vi "FCI_Box_Width.vi"(0 "Image In":T9, 1 "Calibrated Image":T9, 2 "OverlayOptions":T5, 3 "Reference Edge ROI":T12 {"Contours"."Type" items=["No Selection", "Point", "Line", "Rectangle", "Oval", "Polygon", "Freehand Region", "Annulus", "Unused2", "Unused3", "Broken Line", "Freehand Line", "Rotated Rectangle"]}, 4 "Blob Center":cluster{"Center X":dbl, "Center Y":dbl}, 5 "Edge Options Ref ROI":T7={"Edge Polarity"=0, "Kernel Size"=3, "Width"=3, "Minimum Edge Strength"=50.0, "Interpolation Type"=enum."Zero Order", "Data Processing Method"=enum."Average"} {"Edge Polarity" items=["All Edges", "Rising Edges", "Falling Edges"]; "Minimum Edge Strength" format="%.2f"; "Width" step=2; "Kernel Size" step=2}, 7 "error in (no error) 2":errorcluster, 8 "Line Options Ref ROI":T10={"Number of Lines"=1, "Type"=enum."First Edge Rake", "Min. Score"=10.0, "Max. Score"=1000.0, "Orientation"=0.0, "Angle Range"=45.0, "Angle Tolerance"=1.0, "Step Size"=3, "Min. SNR (db)"=0.0, "Min. Points (%)"=25.0, "Hough Iterations"=5} {"Min. Points (%)" min=0.0 max=100.0; "Min. SNR (db)" min=0.0; "Max. Score" min=0.0 max=1024.0; "Min. Score" min=0.0 max=1024.0 step=1.0}, 9 "Search Direction Ref ROI":u32=3, 12 "Edge Options ROI 1":T7={"Edge Polarity"=0, "Kernel Size"=5, "Width"=5, "Minimum Edge Strength"=50.0, "Interpolation Type"=enum."Zero Order", "Data Processing Method"=enum."Average"} {"Edge Polarity" items=["All Edges", "Rising Edges", "Falling Edges"]; "Minimum Edge Strength" format="%.2f"; "Width" step=2; "Kernel Size" step=2}, 13 "Step Size ROI 1":u32=2, 14 "Process ROI 1":T6(ring)=enum."Get First + Last Edge", 15 "Scan Direction ROI 1":u16(ring)=2 items=["Left To Right", "Right To Left", "Top To Bottom", "Bottom To Top"]) -> (18 "Overlay Arrow Lines":T1, 20 "Box Edge Information":T4, 21 "Box Width":sgl, 27 "error IO":errorcluster)   [LabVIEW 2019, in "Algorithm.lvclass"]
uses:
  FrameworkOverrides/Algorithm.lvclass
  <vilib>/vision/Measure.llb/Edge Options.ctl
  <vilib>/vision/Measure.llb/Edge Polarity.ctl
  <vilib>/vision/NI_Vision_Development_Module.lvlib
  <vilib>/vision/Measure.llb/Straight Edge Process.ctl
  <vilib>/vision/Measure.llb/Straight Edge Options.ctl
  <vilib>/vision/Image Controls.llb/IMAQ Image.ctl
panel:
  out "Second Overlay Line":T2
  out "First Overlay Line":T3
  out "Angle (Pixel)":dbl
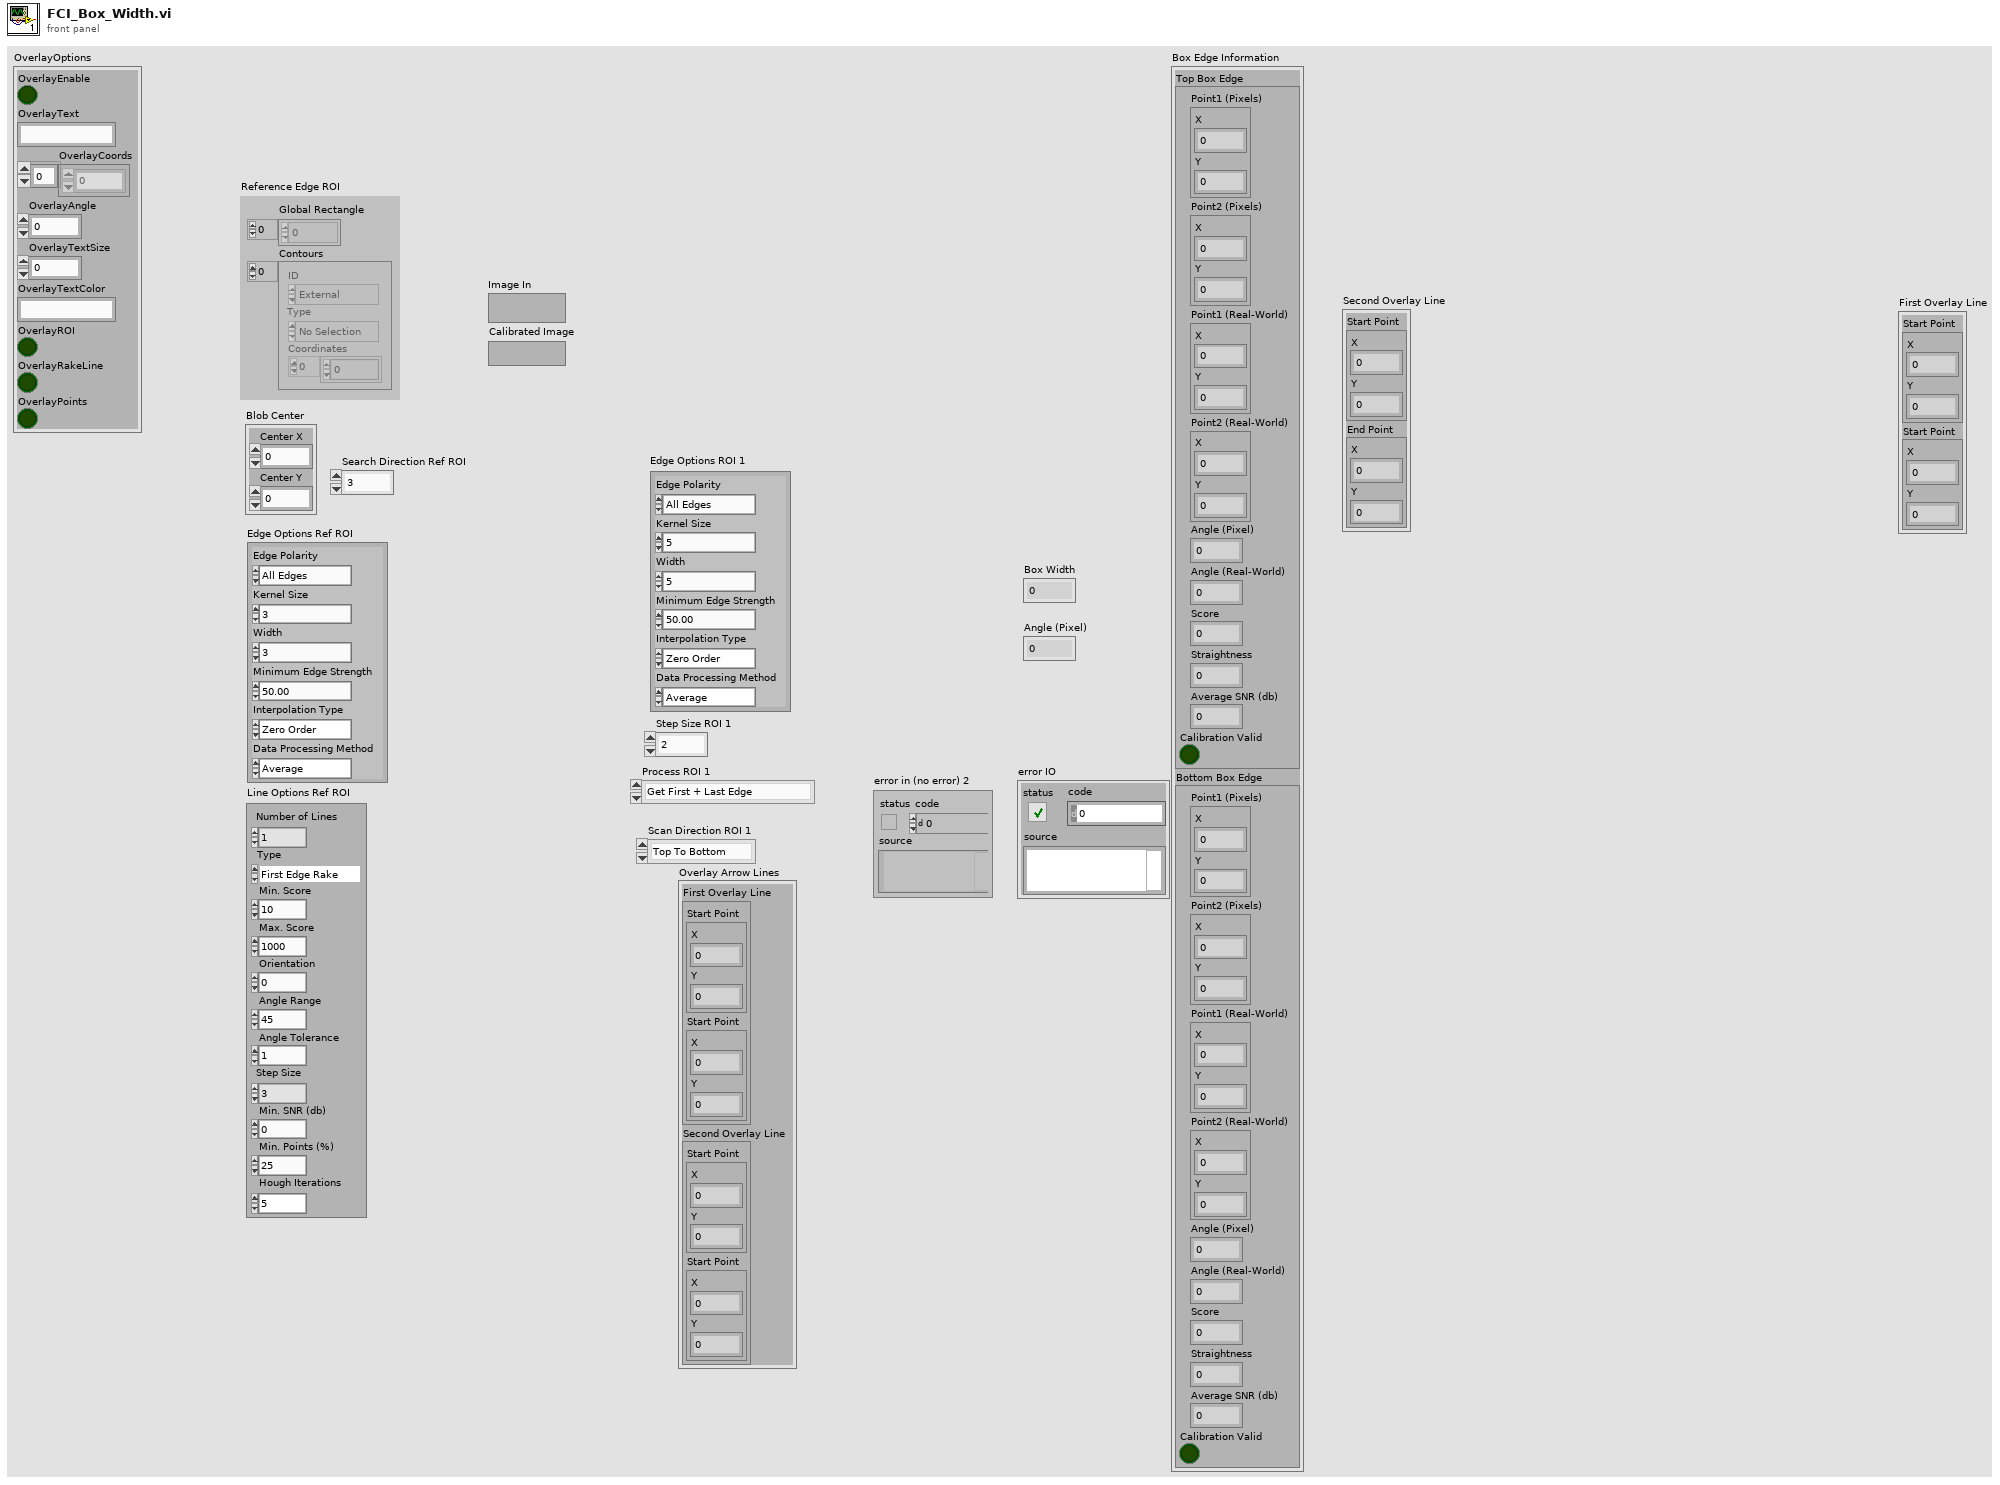
[diagram p1: front panel]
types:
  T1 = cluster{"First Overlay Line ":cluster{"Start Point":cluster{"X":sgl, "Y":sgl}, "Start Point":cluster{"X":sgl, "Y":sgl}}, "Second Overlay Line ":cluster{"Start Point":cluster{"X":sgl, "Y":sgl}, "Start Point":cluster{"X":sgl, "Y":sgl}}}
  T2 = cluster{"Start Point":cluster{"X":sgl, "Y":sgl}, "End Point":cluster{"X":sgl, "Y":sgl}}
  T3 = cluster{"Start Point":cluster{"X":sgl, "Y":sgl}, "Start Point":cluster{"X":sgl, "Y":sgl}}
  T4 = cluster{"Top Box Edge":cluster{"Point1 (Pixels)":cluster{"X":sgl, "Y":sgl}, "Point2 (Pixels)":cluster{"X":sgl, "Y":sgl}, "Point1 (Real-World)":cluster{"X":sgl, "Y":sgl}, "Point2 (Real-World)":cluster{"X":sgl, "Y":sgl}, "Angle (Pixel)":dbl, "Angle (Real-World)":dbl, "Score":dbl, "Straightness":dbl, "Average SNR (db)":dbl, "Calibration Valid":bool}, "Bottom Box Edge":cluster{"Point1 (Pixels)":cluster{"X":sgl, "Y":sgl}, "Point2 (Pixels)":cluster{"X":sgl, "Y":sgl}, "Point1 (Real-World)":cluster{"X":sgl, "Y":sgl}, "Point2 (Real-World)":cluster{"X":sgl, "Y":sgl}, "Angle (Pixel)":dbl, "Angle (Real-World)":dbl, "Score":dbl, "Straightness":dbl, "Average SNR (db)":dbl, "Calibration Valid":bool}}
  T5 = cluster{"OverlayEnable":bool, "OverlayText":string, "OverlayCoords":i32[], "OverlayAngle":i32, "OverlayTextSize":i32, "OverlayTextColor":string, "OverlayROI":bool, "OverlayRakeLine":bool, "OverlayPoints":bool}
  T6 = enum16{"Get First Edge", "Get First + Last Edge", "Get All Edges", "Get Best Edge"}
  T7 = typedef "Edge Options.ctl" = cluster{"Edge Polarity":T8, "Kernel Size":u32, "Width":u32, "Minimum Edge Strength":sgl, "Interpolation Type":enum32{"Zero Order", "Bilinear", "Quadratic", "Cubic", "Bilinear Fixed"}, "Data Processing Method":enum32{"Average", "Median"}}
  T8 = typedef "Edge Polarity.ctl" = u32
  T9 = typedef "IMAQ Image.ctl" = refnum<image>
  T10 = typedef "Straight Edge Options.ctl" = cluster{"Number of Lines":i32, "Type":T11, "Min. Score":dbl, "Max. Score":dbl, "Orientation":dbl, "Angle Range":dbl, "Angle Tolerance":dbl, "Step Size":u32, "Min. SNR (db)":dbl, "Min. Points (%)":dbl, "Hough Iterations":i32}
  T11 = typedef "Straight Edge Process.ctl" = enum32{"First Edge Rake", "Best Edge Rake", "Hough Edge Rake", "First Edge Projection", "Best Edge Projection"}
  T12 = typedef "ROI Descriptor" = cluster{"Global Rectangle":i32[], "Contours":cluster{"ID":enum32{"External", "Internal"}, "Type":u32, "Coordinates":i32[]}[]}
  T13 = cluster{"Search Direction":u32, "Edge Options":T7, "Show Search Area":bool, "Show Search Lines":bool, "Show Edges Found":bool, "Show Result":bool, "Search Area Color":u32, "Search Lines Color":u32, "Edge Locations Color":u32, "Result Color":u32, "Overlay Group Name":string}
  T14 = cluster{"Left":i32, "Top":i32, "Right":i32, "Bottom":i32, "Angle":dbl}
  T15 = cluster{"Left":dbl, "Top":dbl, "Right":dbl, "Bottom":dbl, "Angle":dbl}
  T16 = typedef "IMAQ Rectangle" = cluster{"Left":i32, "Top":i32, "Right":i32, "Bottom":i32, "Rotation":dbl}
  T17 = cluster{"Point1 (Pixels)":cluster{"X":sgl, "Y":sgl}, "Point2 (Pixels)":cluster{"X":sgl, "Y":sgl}, "Point1 (Real-World)":cluster{"X":sgl, "Y":sgl}, "Point2 (Real-World)":cluster{"X":sgl, "Y":sgl}, "Angle (Pixel)":dbl, "Angle (Real-World)":dbl, "Score":dbl, "Straightness":dbl, "Average SNR (db)":dbl, "Calibration Valid":bool}[]
  T18 = cluster{"Point1 (Pixels)":cluster{"X":sgl, "Y":sgl}, "Point2 (Pixels)":cluster{"X":sgl, "Y":sgl}, "Point1 (Real-World)":cluster{"X":sgl, "Y":sgl}, "Point2 (Real-World)":cluster{"X":sgl, "Y":sgl}, "Angle (Pixel)":dbl, "Angle (Real-World)":dbl, "Score":dbl, "Straightness":dbl, "Average SNR (db)":dbl, "Calibration Valid":bool}
  T19 = typedef "Edge New.ctl" = cluster{"Location (Pixel)":cluster{"X":sgl, "Y":sgl}, "Location (Real-World)":cluster{"X":sgl, "Y":sgl}, "Distance (Pixel)":dbl, "Distance (Real-World)":dbl, "Strength":dbl, "Noise":dbl, "Rising?":bool}
  T20 = typedef "Search Line.ctl" = cluster{"Start Point":cluster{"X":sgl, "Y":sgl}, "End Point":cluster{"X":sgl, "Y":sgl}, "Edge Info":T19[], "Edge Map":dbl[], "Calibration Valid":bool}
  T21 = cluster{"Start Point":cluster{"X":sgl, "Y":sgl}, "Location (Pixel)":cluster{"X":sgl, "Y":sgl}}
  T22 = cluster{"Location (Pixel)":cluster{"X":sgl, "Y":sgl}, "End Point":cluster{"X":sgl, "Y":sgl}}
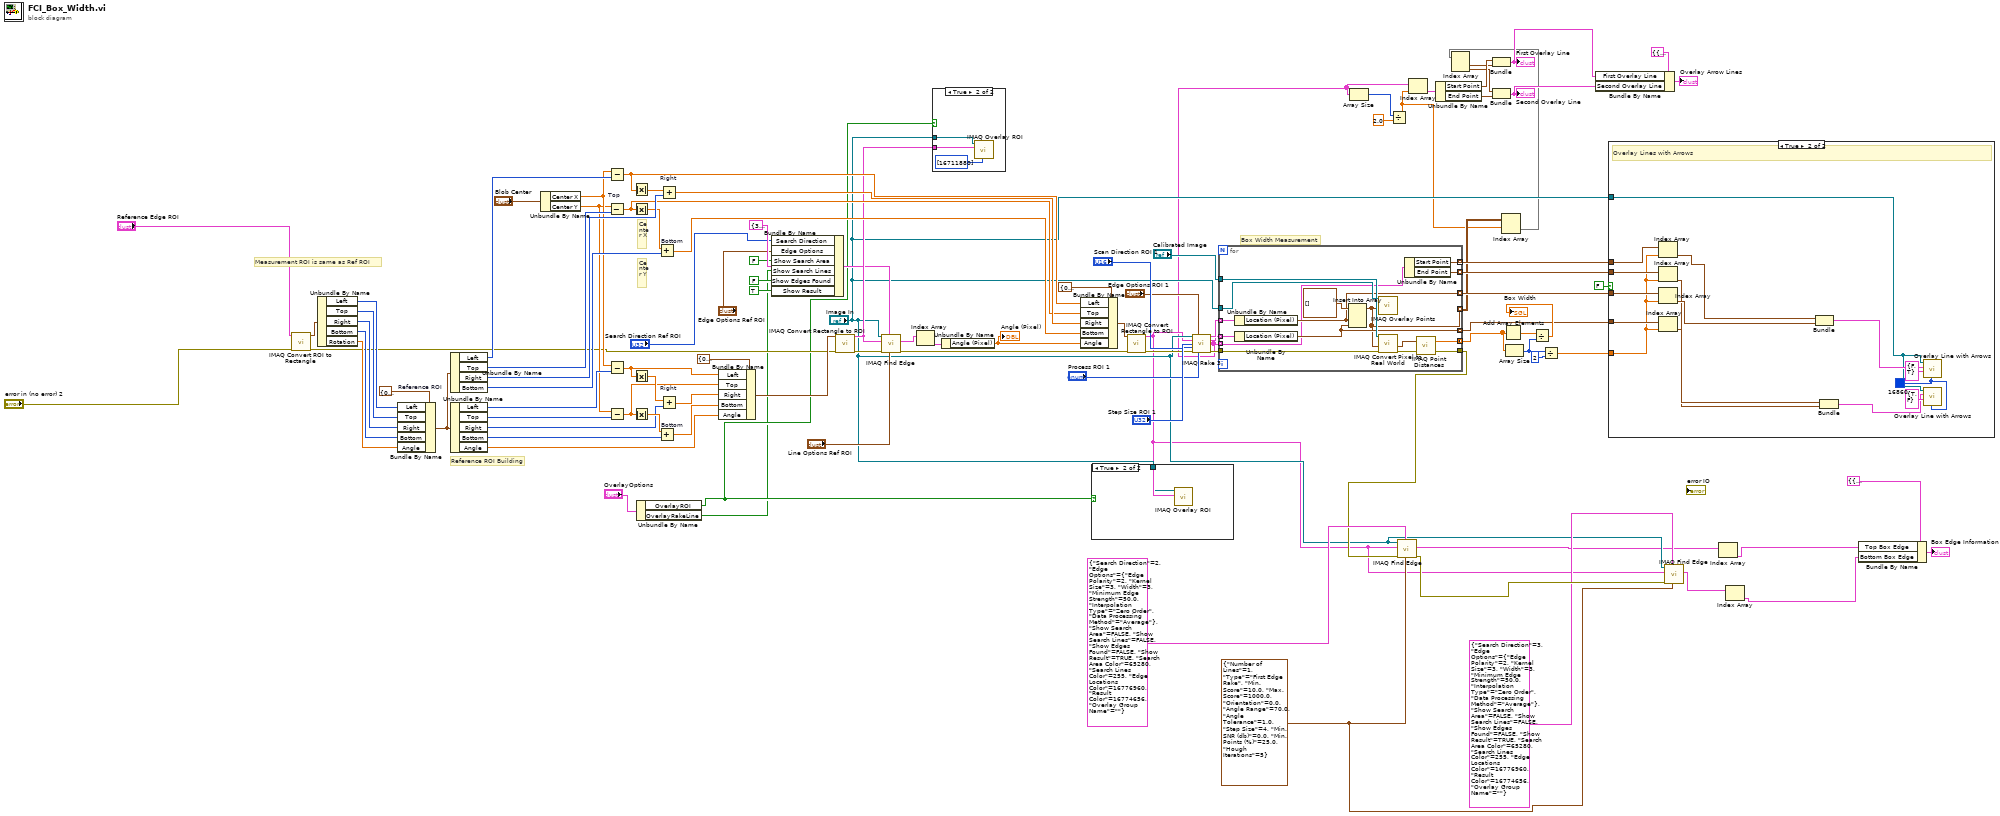
[diagram p0: block diagram]
diagram:
  w23 = T10 {"Number of Lines"=1, "Type"=enum."First Edge Rake", "Min. Score"=10.0, "Max. Score"=1000.0, "Orientation"=0.0, "Angle Range"=70.0, "Angle Tolerance"=1.0, "Step Size"=4, "Min. SNR (db)"=0.0, "Min. Points (%)"=25.0, "Hough Iterations"=5} ("Line Fit Options")
  # "Measurement ROI is same as Ref ROI"
  # "Box Width Measurement"
  # "Reference ROI Building"
  # "Center Y"
  # "Center X"
  n1 = call "IMAQ Convert ROI to Rectangle"("error in (no error)"="error in (no error) 2", "ROI Descriptor"="Reference Edge ROI") -> ("error out"=w41:errorcluster, "Rectangle"=w55:T16)  [unwired: 7 in]
  n2 = Unbundle By Name(w55) -> ("Left"=w53:i32, "Top"=w52:i32, "Right"=w51:i32, "Bottom"=w50:i32, "Rotation"=w54:dbl)
  n3 = Bundle By Name "Reference ROI"(cluster=T14 {"Left"=0, "Top"=0, "Right"=0, "Bottom"=0, "Angle"=0.0} ("input cluster"), "Left"=w53, "Top"=w52, "Right"=w51, "Bottom"=w50, "Angle"=w54) -> (w60:T14)
  n4 = Unbundle By Name(w60) -> ("Left"=w92:i32, "Top"=w91:i32, "Right"=w90:i32, "Bottom"=w89:i32)
  n5 = Unbundle By Name(w60) -> ("Left"=w88:i32, "Top"=w87:i32, "Right"=w86:i32, "Bottom"=w85:i32, "Angle"=w84:dbl)
  n6 = Unbundle By Name("Blob Center") -> ("Center X"=w58:dbl, "Center Y"=w57:dbl)
  n7 = Subtract "Top"(x=w57, y=w91) -> (x-y=w67:dbl)
  n8 = Subtract(x=w58, y=w92) -> (x-y=w102:dbl)
  n9 = Subtract(x=w58, y=w88) -> (x-y=w96:dbl)
  n10 = Subtract(x=w57, y=w87) -> (x-y=w95:dbl)
  n11 = Absolute Value(x=w102) -> (abs(x)=w104:dbl)
  n12 = Absolute Value(x=w67) -> (abs(x)=w68:dbl)
  n13 = Absolute Value(x=w96) -> (abs(x)=w99:dbl)
  n14 = Absolute Value(x=w95) -> (abs(x)=w98:dbl)
  n15 = Unbundle By Name("OverlayOptions") -> ("OverlayROI"=w30:bool, "OverlayRakeLine"=w29:bool)
  n16 = Add "Bottom"(x=w68, y=w89) -> (x+y=w100:dbl)
  n17 = Add "Bottom"(x=w98, y=w85) -> (x+y=w93:dbl)
  n18 = Add "Right"(x=w104, y=w90) -> (x+y=w101:dbl)
  n19 = Add "Right"(x=w99, y=w86) -> (x+y=w94:dbl)
  n20 = Bundle By Name(cluster=T15 {"Left"=0.0, "Top"=0.0, "Right"=0.0, "Bottom"=0.0, "Angle"=0.0} ("input cluster"), "Left"=w96, "Top"=w95, "Right"=w94, "Bottom"=w93, "Angle"=w84) -> (w71:T15)
  n21 = Bundle By Name(cluster=T13 {"Search Direction"=3, "Edge Options"={"Edge Polarity"=0, "Kernel Size"=3, "Width"=3, "Minimum Edge Strength"=50.0, "Interpolation Type"=enum."Zero Order", "Data Processing Method"=enum."Average"}, "Show Search Area"=FALSE, "Show Search Lines"=FALSE, "Show Edges Found"=FALSE, "Show Result"=TRUE, "Search Area Color"=16860, "Search Lines Color"=255, "Edge Locations Color"=16776960, "Result Color"=16711680, "Overlay Group Name"=""} ("Options"), "Search Direction"="Search Direction Ref ROI", "Edge Options"="Edge Options Ref ROI", "Show Search Area"=FALSE, "Show Search Lines"=w29, "Show Edges Found"=FALSE, "Show Result"=TRUE) -> (w43:T13)
  n22 = call "IMAQ Convert Rectangle to ROI"("error in (no error)"=w41, "Rectangle"=w71) -> ("error out"=w83:errorcluster, "ROI Descriptor"=w65:T12)  [unwired: 7 in]
  n23 = call "IMAQ Find Edge"("Line Fit Options"="Line Options Ref ROI", "Options"=w43, "error in (no error)"=w83, "ROI Descriptor"=w65, "Image"="Image In") -> ("error out"=w64:errorcluster, "Straight Edges"=w81:T17)  [unwired: 3 in, 2 out]
  n24 = Index Array(array=w81) -> (element=w80:T18)  [unwired: 1 in]
  n25 = case shown="True" w30 {
    tunnel: w65 -> [_ w107]
    tunnel: "Image In" -> [_ w105]
    frame False {
    }
    frame True {
      n26 = call "IMAQ Overlay ROI"("Colors (Green)"=u32[] [16711880], "ROI Descriptor"=w107, "Image"=w105) -> ()  [unwired: 7 in, 2 out]
    }
  }
  n27 = Unbundle By Name(w80) -> ("Angle (Pixel)"=w61:dbl)
  "Angle (Pixel)" <- w61
  n28 = Bundle By Name(cluster=T15 {"Left"=0.0, "Top"=0.0, "Right"=0.0, "Bottom"=0.0, "Angle"=0.0} ("input cluster"), "Left"=w102, "Top"=w67, "Right"=w101, "Bottom"=w100, "Angle"=w61) -> (w70:T15)
  n29 = call "IMAQ Convert Rectangle to ROI"("error in (no error)"=w64, "Rectangle"=w70) -> ("error out"=w63:errorcluster, "ROI Descriptor"=w22:T12)  [unwired: 7 in]
  n30 = case shown="True" w30 {
    tunnel: w22 -> [_ w109]
    tunnel: "Image In" -> [_ w108]
    frame False {
    }
    frame True {
      n31 = call "IMAQ Overlay ROI"("ROI Descriptor"=w109, "Image"=w108) -> ()  [unwired: 8 in, 2 out]
    }
  }
  n32 = call "IMAQ Rake 3"("Image"="Image In", "Edge Options"="Edge Options ROI 1", "ROI Descriptor"=w22, "Step Size"="Step Size ROI 1", "Scan Direction"="Scan Direction ROI 1", "error in (no error)"=w63, "Process"="Process ROI 1") -> ("First Edges"=w75:T19[], "Last Edges"=w69:T19[], "Search Lines"=w5:T20[], "error out"=w62:errorcluster)  [unwired: 5 in]
  n33 = for {
    tunnel: w75 -> [w125] mode=indexing
    tunnel: w69 -> [w124] mode=indexing
    tunnel: [w122] -> w74 mode=concatenating
    tunnel: "Image In" -> [w121]
    tunnel: w62 -> [w119]
    tunnel: [w120] -> w27
    tunnel: w5 -> [w113] mode=indexing
    tunnel: "Calibrated Image" -> [w116]
    tunnel: [w115] -> w37 mode=indexing
    tunnel: [w114] -> w36 mode=indexing
    tunnel: [w112] -> w35 mode=indexing
    tunnel: [w111] -> w34 mode=indexing
    tunnel: [w110] -> w4 mode=indexing
    n34 = Unbundle By Name(w125) -> ("Location (Pixel)"=w115:cluster{"X":sgl, "Y":sgl})
    n35 = Unbundle By Name(w124) -> ("Location (Pixel)"=w114:cluster{"X":sgl, "Y":sgl})
    n36 = Insert Into Array(array=cluster{"X":sgl, "Y":sgl}[] [], new element #1=w115, new element #2=w114) -> (w110:cluster{"X":sgl, "Y":sgl}[])  [unwired: 1 in]
    n37 = call "IMAQ Overlay Points"("Array of Points"=w110, "Image"=w121) -> ()  [unwired: 8 in, 2 out]
    n38 = call "IMAQ Convert Pixel to Real World"("error in (no error)"=w119, "Array of Pixel Coordinates"=w110, "Calibrated Image"=w116) -> ("error out"=w117:errorcluster, "Array of Real World Coordinates"=w118:cluster{"X":sgl, "Y":sgl}[])  [unwired: 3 in, 4 out]
    n39 = Unbundle By Name(w113) -> ("Start Point"=w112:cluster{"X":sgl, "Y":sgl}, "End Point"=w111:cluster{"X":sgl, "Y":sgl})
    n40 = call "IMAQ Point Distances"("Points"=w118, "error in (no error)"=w117) -> ("Distances"=w122:sgl[], "error out"=w120:errorcluster)  [unwired: 3 in]
  }
  n41 = Array Size(array=w5) -> (size(s)=w6:i32)
  n42 = Divide(x=w6, y=2.0) -> (x/y=w3:dbl)
  n43 = call "IMAQ Find Edge"("Line Fit Options"=w23, "Options"=T13 {"Search Direction"=2, "Edge Options"={"Edge Polarity"=2, "Kernel Size"=3, "Width"=3, "Minimum Edge Strength"=50.0, "Interpolation Type"=enum."Zero Order", "Data Processing Method"=enum."Average"}, "Show Search Area"=FALSE, "Show Search Lines"=FALSE, "Show Edges Found"=FALSE, "Show Result"=TRUE, "Search Area Color"=65280, "Search Lines Color"=255, "Edge Locations Color"=16776960, "Result Color"=16774656, "Overlay Group Name"=""}, "error in (no error)"=w27, "ROI Descriptor"=w22, "Image"="Image In") -> ("error out"=w26:errorcluster, "Straight Edges"=w21:T17)  [unwired: 3 in, 2 out]
  n44 = Index Array(array=w5, index=w3) -> (element=w15:T20)
  n45 = Unbundle By Name(w15) -> ("Start Point"=w14:cluster{"X":sgl, "Y":sgl}, "End Point"=w11:cluster{"X":sgl, "Y":sgl})
  n46 = Index Array(array=w4, index (row)=w3) -> (element=w2:cluster{"X":sgl, "Y":sgl}[])  [unwired: 1 in]
  n47 = Index Array(array=w2) -> (element #1=w13:cluster{"X":sgl, "Y":sgl}, element #2=w12:cluster{"X":sgl, "Y":sgl})  [unwired: 2 in]
  n48 = Bundle("Start Point"=w14, "Location (Pixel)"=w13) -> (w9:T21)  [unwired: 1 in]
  "First Overlay Line" <- w9
  n49 = Bundle("Location (Pixel)"=w12, "End Point"=w11) -> (w8:T22)  [unwired: 1 in]
  "Second Overlay Line" <- w8
  n50 = Add Array Elements(numeric array=w74) -> (sum=w73:sgl)
  n51 = Array Size(array=w74) -> (size(s)=w39:i32)
  n52 = Divide(x=w73, y=w39) -> (x/y=→"Box Width":sgl)
  n53 = Divide(x=w39, y=2) -> (x/y=w33:dbl)
  n54 = Bundle By Name(cluster=T1 {"First Overlay Line "={"Start Point"={"X"=0.0, "Y"=0.0}, "Start Point"={"X"=0.0, "Y"=0.0}}, "Second Overlay Line "={"Start Point"={"X"=0.0, "Y"=0.0}, "Start Point"={"X"=0.0, "Y"=0.0}}}, "First Overlay Line"=w9, "Second Overlay Line"=w8) -> (→"Overlay Arrow Lines":T1)
  n55 = case shown="True" FALSE {
    tunnel: w37 -> [_ w140]
    tunnel: w36 -> [_ w139]
    tunnel: w35 -> [_ w138]
    tunnel: w34 -> [_ w137]
    tunnel: w33 -> [_ w136]
    tunnel: "Image In" -> [_ w126]
    frame False {
    }
    frame True {
      w133 = u32 16860 ("Color")
      # "Overlay Lines with Arrows"
      n56 = Index Array(array=w138, index=w136) -> (element=w130:cluster{"X":sgl, "Y":sgl})
      n57 = Index Array(array=w137, index=w136) -> (element=w127:cluster{"X":sgl, "Y":sgl})
      n58 = Index Array(array=w140, index=w136) -> (element=w129:cluster{"X":sgl, "Y":sgl})
      n59 = Index Array(array=w139, index=w136) -> (element=w128:cluster{"X":sgl, "Y":sgl})
      n60 = Bundle("Start Point"=w130, "Location (Pixel)"=w129) -> (w131:T21)  [unwired: 1 in]
      n61 = Bundle("Location (Pixel)"=w128, "End Point"=w127) -> (w132:T22)  [unwired: 1 in]
      n62 = call <vilib>:"Overlay Line with Arrows.vi"("Color"=w133, "Arrows"=cluster{"Start point":bool, "End point":bool} {"Start point"=FALSE, "End point"=TRUE}, "Line Coordinates"=w131, "Image In"=w126) -> ()  [unwired: 6 in, 2 out]
      n63 = call <vilib>:"Overlay Line with Arrows.vi"("Color"=w133, "Arrows"=cluster{"Start point":bool, "End point":bool} {"Start point"=TRUE, "End point"=FALSE}, "Line Coordinates"=w132, "Image In"=w126) -> ()  [unwired: 6 in, 2 out]
    }
  }
  n64 = call "IMAQ Find Edge"("Line Fit Options"=w23, "Options"=T13 {"Search Direction"=3, "Edge Options"={"Edge Polarity"=2, "Kernel Size"=3, "Width"=3, "Minimum Edge Strength"=50.0, "Interpolation Type"=enum."Zero Order", "Data Processing Method"=enum."Average"}, "Show Search Area"=FALSE, "Show Search Lines"=FALSE, "Show Edges Found"=FALSE, "Show Result"=TRUE, "Search Area Color"=65280, "Search Lines Color"=255, "Edge Locations Color"=16776960, "Result Color"=16774656, "Overlay Group Name"=""}, "error in (no error)"=w26, "ROI Descriptor"=w22, "Image"="Image In") -> ("Straight Edges"=w20:T17)  [unwired: 3 in, 3 out]
  n65 = Index Array(array=w21) -> (element=w18:T18)  [unwired: 1 in]
  n66 = Index Array(array=w20) -> (element=w17:T18)  [unwired: 1 in]
  n67 = Bundle By Name(cluster=T4 {"Top Box Edge"={"Point1 (Pixels)"={"X"=0.0, "Y"=0.0}, "Point2 (Pixels)"={"X"=0.0, "Y"=0.0}, "Point1 (Real-World)"={"X"=0.0, "Y"=0.0}, "Point2 (Real-World)"={"X"=0.0, "Y"=0.0}, "Angle (Pixel)"=0.0, "Angle (Real-World)"=0.0, "Score"=0.0, "Straightness"=0.0, "Average SNR (db)"=0.0, "Calibration Valid"=FALSE}, "Bottom Box Edge"={"Point1 (Pixels)"={"X"=0.0, "Y"=0.0}, "Point2 (Pixels)"={"X"=0.0, "Y"=0.0}, "Point1 (Real-World)"={"X"=0.0, "Y"=0.0}, "Point2 (Real-World)"={"X"=0.0, "Y"=0.0}, "Angle (Pixel)"=0.0, "Angle (Real-World)"=0.0, "Score"=0.0, "Straightness"=0.0, "Average SNR (db)"=0.0, "Calibration Valid"=FALSE}}, "Top Box Edge"=w18, "Bottom Box Edge"=w17) -> (→"Box Edge Information":T4)
